vi "CSM - Async Start Group of CSMs.vi"(4 "Information":refnum<vi>, 5 "Prototypes":refnum<vi>[](array[refnum]), 6 "error in (no error)":errorcluster, 7 "interval(50ms)":u32=50, 8 "Wait for Module Ready?(T)":bool=TRUE, 9 "Module List":cluster{"ModuleName":string, "Index":i32}[](array[cluster])) -> (0 "error out":errorcluster)   [LabVIEW 2020, in "CSMStand(Lite).lvlib"]
uses:
  CSMStand(Lite).lvlib
  <userlib>/_NEVSTOP/Communicable State Machine(CSM)/Communicable State Machine.lvlib
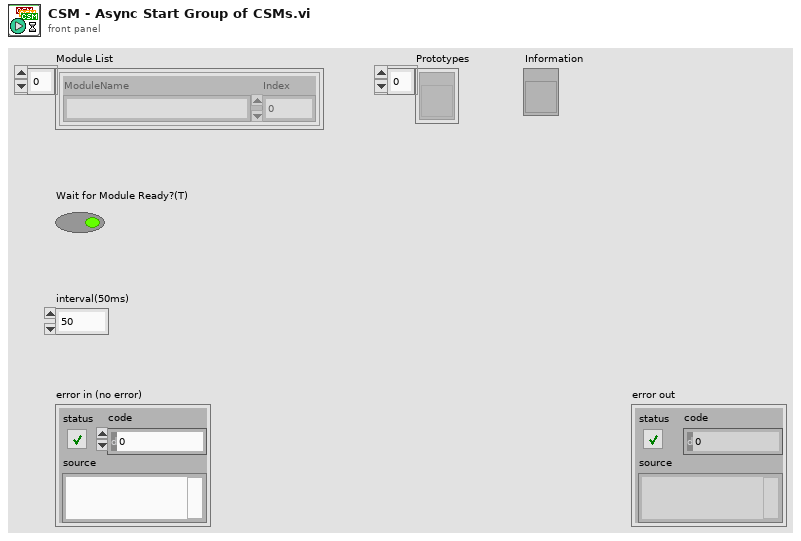
[diagram p1: front panel]
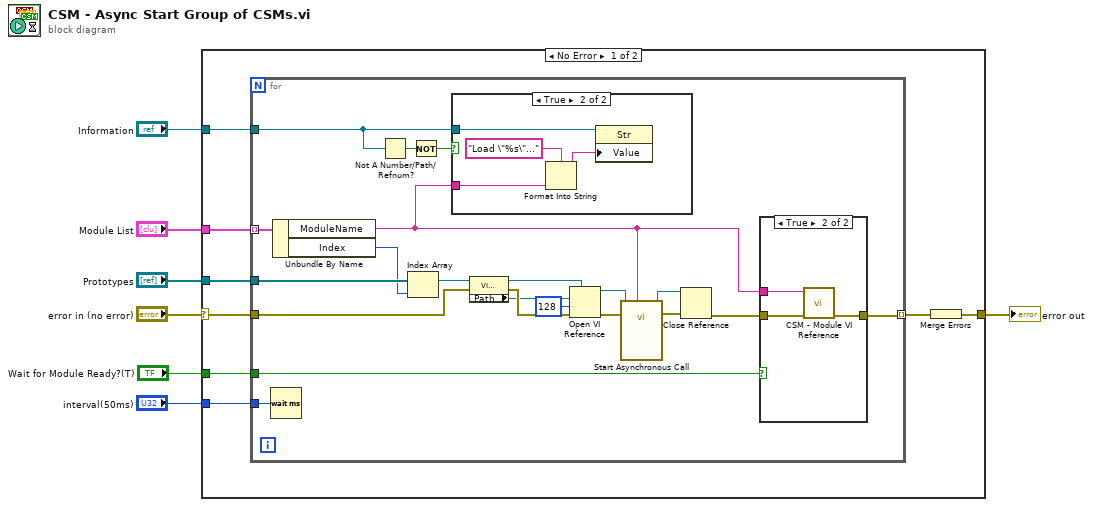
[diagram p0: block diagram]
diagram:
  n1 = case shown="No Error" "error in (no error)" {
    selector: "error in (no error)" -> [w12 w45]
    tunnel: "Module List" -> [w14 _]
    tunnel: "Prototypes" -> [w13 _]
    tunnel: "interval(50ms)" -> [w11 _]
    tunnel: "Information" -> [w10 _]
    tunnel: "Wait for Module Ready?(T)" -> [w9 _]
    tunnel: [w8 w45] -> w1
    frame No Error {
      n2 = for {
        tunnel: w13 -> [w26]
        tunnel: w14 -> [w25] mode=indexing
        tunnel: w11 -> [w22]
        tunnel: w10 -> [w21]
        tunnel: w9 -> [w16]
        tunnel: w12 -> [w28]
        tunnel: [w18] -> w15 mode=indexing
        n3 = Wait (ms)(milliseconds to wait=w22) -> ()  [unwired: 1 out]
        n4 = Unbundle By Name(w25) -> ("ModuleName"=w17:string, "Index"=w23:i32)
        n5 = Not A Number/Path/Refnum?(number/path/refnum=w21) -> (NaN/Path/Refnum?=w19:bool)
        n6 = Index Array(array=w26, index=w23) -> (element=w24:refnum<vi>)
        n7 = Not(x=w19) -> (.not. x?=w20:bool)
        n8 = case shown="True" w20 {
          tunnel: w21 -> [_ w44]
          tunnel: w17 -> [_ w42]
          frame False {
          }
          frame True {
            n9 = Format Into String(format string="Load \"%s\"...", w42) -> (resulting string=w41:string)  [unwired: 2 in, 1 out]
            n10 = property class="Str"(reference=w44, "Value"=w41) -> ()  [unwired: 1 in, 2 out]
          }
        }
        n11 = property class="VI (strict)"(reference=w24, error in=w28) -> (reference out=w33:refnum<vi>, error out=w31:errorcluster, "Path"=w30:path)
        n12 = Open VI Reference(type specifier VI Refnum (for type only)=w33, vi path=w30, options=128, error in (no error)=w31) -> (vi reference=w32:refnum<vi>, error out=w29:errorcluster)  [unwired: 2 in]
        n13 = call-by-ref "Start Asynchronous Call"(reference=w32, error in=w29, "Name(\"\" to use uuid)"=w17) -> (reference out=w35:refnum<vi>, error out=w34:errorcluster)  [unwired: 11 in]
        n14 = Close Reference(reference=w35, error in (no error)=w34) -> (error out=w27:errorcluster)
        n15 = case shown="True" w16 {
          tunnel: w27 -> [w37 w40]
          tunnel: [w37 w39] -> w18
          tunnel: w17 -> [_ w38]
          frame False {
          }
          frame True {
            n16 = call <userlib>:"CSM - Module VI Reference.vi"("error in (no error)"=w40, "CSM Name"=w38) -> ("error out"=w39:errorcluster)  [unwired: 8 in, 1 out]
          }
        }
      }
      n17 = Merge Errors(w15) -> (w8:errorcluster)
    }
    frame Error {
    }
  }
  "error out" <- w1
